vi "besLinearFiIntoExceltvi.vi"() -> ()   [LabVIEW 2015]
uses:
  <vilib>/Analysis/6fits.llb/Curve Fitting Criteria.ctl
  <vilib>/Utility/file.llb/Write Delimited Spreadsheet (string).vi
  <vilib>/Analysis/NI_AALPro.lvlib
panel:
  in  "X Data":dbl[](array[numeric])=[0.0, 2.0, 4.0, 6.0, 8.0, 12.0, 14.0]
  in  "Y Data":dbl[](array[numeric])=[12.0, 25.0, 37.0, 47.0, 66.0, 87.0, 102.0]
  out "slope":dbl
  out "intercept":dbl
  out "error":i32
  in  "method":T1 items=["Least Square", "Least Absolute Residual", "Bisquare"]
  out "XY Graph":T2(graph)
  in  "Table":string[][](table)
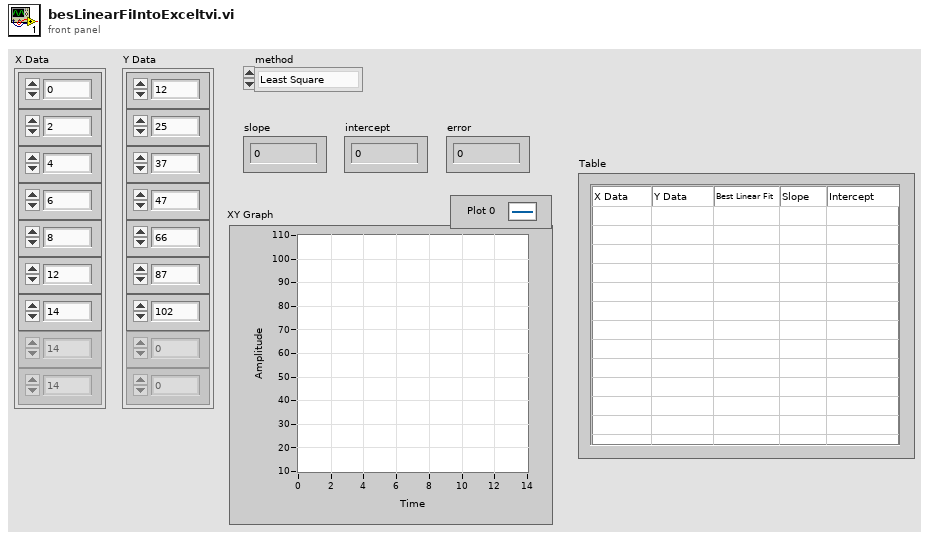
[diagram p1: front panel]
types:
  T1 = typedef "NI_AALPro.lvlib/Curve Fitting Criteria.ctl" = u16
  T2 = cluster{"X Data ":dbl[], "Best Linear Fit":dbl[]}[]
  T3 = cluster{"X Data ":dbl[], "Best Linear Fit":dbl[]}
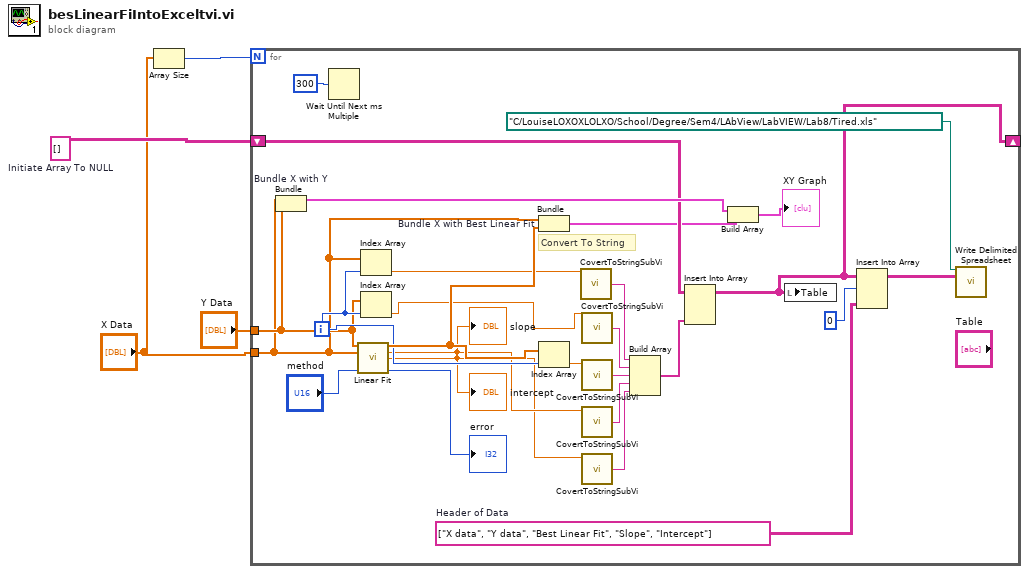
[diagram p0: block diagram]
diagram:
  w4 = string[][] []  # Initiate Array To NULL
  n1 = Array Size(array="X Data") -> (size(s)=w1:i32)
  n2 = for {
    N: w1 -> [_]
    shift-right: [w6] -> _
    shift-left: w4 -> [w26]
    tunnel: "Y Data" -> [w10]
    tunnel: "X Data" -> [w9]
    i -> [w24]
    w8 = string[][] [["X data", "Y data", "Best Linear Fit", "Slope", "Intercept"]]  # Header of Data
    # "Convert To String"
    n3 = Bundle "Bundle X with Y"("X Data"=w9, "Y Data"=w10) -> (w28:cluster{"X Data ":dbl[], "Y Data ":dbl[]})  [unwired: 1 in]
    n4 = Wait Until Next ms Multiple(millisecond multiple=u32 300) -> ()  [unwired: 1 out]
    n5 = call <vilib>:"Linear Fit.vi"("Y"=w10, "X"=w9, "method"="method") -> ("Best Linear Fit"=w27:dbl[], "slope"=w16:dbl, "intercept"=w14:dbl, "error"=→"error":i32)  [unwired: 8 in, 1 out]
    "slope" <- w16
    "intercept" <- w14
    n6 = Index Array(array=w9, index=w24) -> (element=w22:dbl)
    n7 = Index Array(array=w10, index=w24) -> (element=w20:dbl)
    n8 = Bundle "Bundle X with Best Linear Fit"("X Data"=w9, "Best Linear Fit"=w27) -> (w12:T3)  [unwired: 1 in]
    n9 = Index Array(array=w27, index=w24) -> (element=w18:dbl)
    n10 = call "CovertToStringSubVi.vi"("input"=w22) -> ("resulting string"=w21:string)  [unwired: 4 in]
    n11 = call "CovertToStringSubVi.vi"("input"=w20) -> ("resulting string"=w19:string)  [unwired: 4 in]
    n12 = call "CovertToStringSubVi.vi"("input"=w18) -> ("resulting string"=w17:string)  [unwired: 4 in]
    n13 = call "CovertToStringSubVi.vi"("input"=w16) -> ("resulting string"=w15:string)  [unwired: 4 in]
    n14 = call "CovertToStringSubVi.vi"("input"=w14) -> ("resulting string"=w13:string)  [unwired: 4 in]
    n15 = Build Array(w21, w19, w17, w15, w13) -> (w23:string[])
    n16 = Insert Into Array "Insert Into Array"(array=w26, new element=w23) -> (w6:string[][])  [unwired: 2 in]
    n17 = Build Array(w28, w12) -> (→"XY Graph":T2)
    n18 = local write "Table"(w6) -> ()
    n19 = Insert Into Array "Insert Into Array"(array=w6, index (row)=0, new element=w8) -> (w5:string[][])  [unwired: 1 in]
    n20 = call-poly <vilib>:"Write Delimited Spreadsheet.vi"("file path (dialog if empty)"=path "C:/LouiseLOXOXLOLXO/School/Degree/Sem4/LAbView/LabVIEW/Lab8/Tired.xls", "2D data"=w5) -> ()  [unwired: 12 in, 2 out]
  }
